vi "main elapsed time.vi"() -> ()   [LabVIEW 2019]
uses:
  Controls/Estats.ctl
panel:
  out "Numeric":i32
  in  "stop":bool
  out "Boolean":bool
  # "fixar-se en la velocitat d'execució ara"
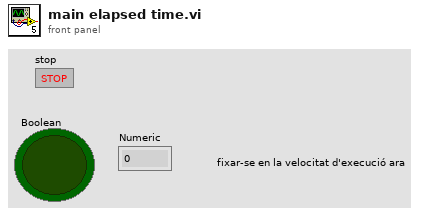
[diagram p1: front panel]
types:
  T1 = typedef "Estats.ctl" = enum16{"inicialitza", "Estat1", "Estat2"}
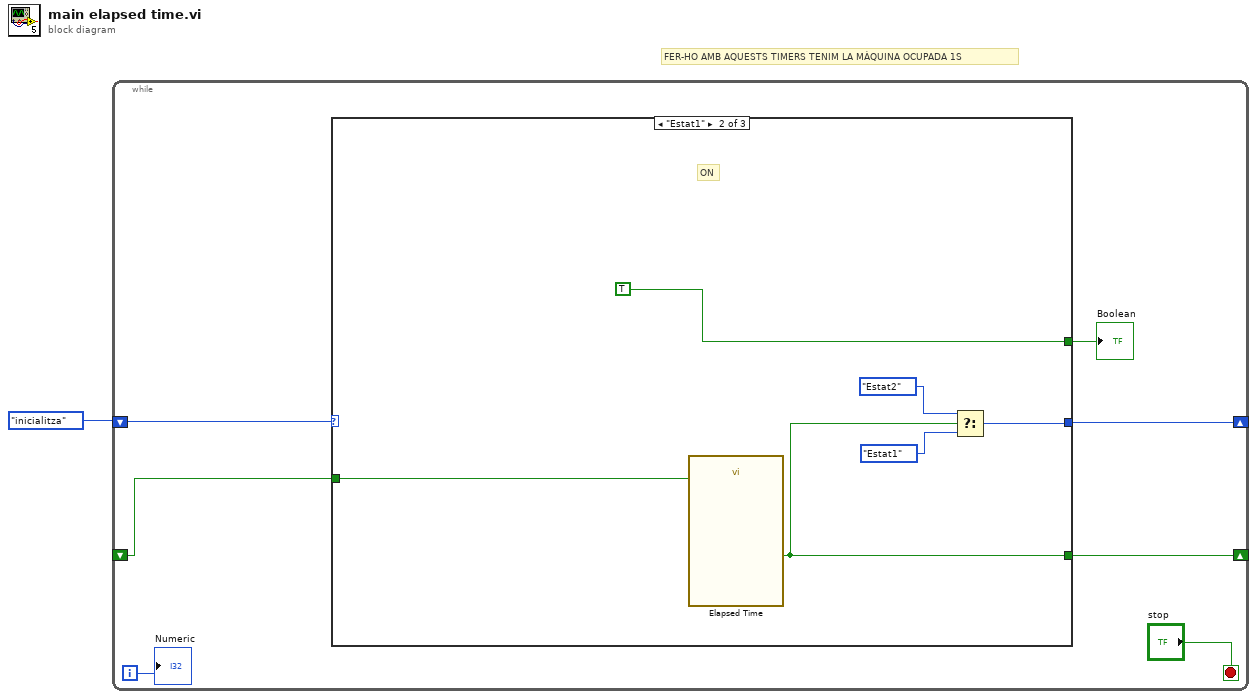
[diagram p0: block diagram]
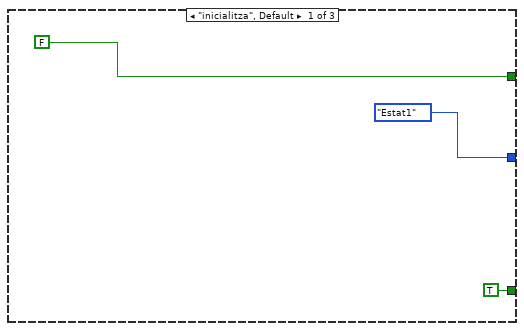
[diagram p2: hidden frame]
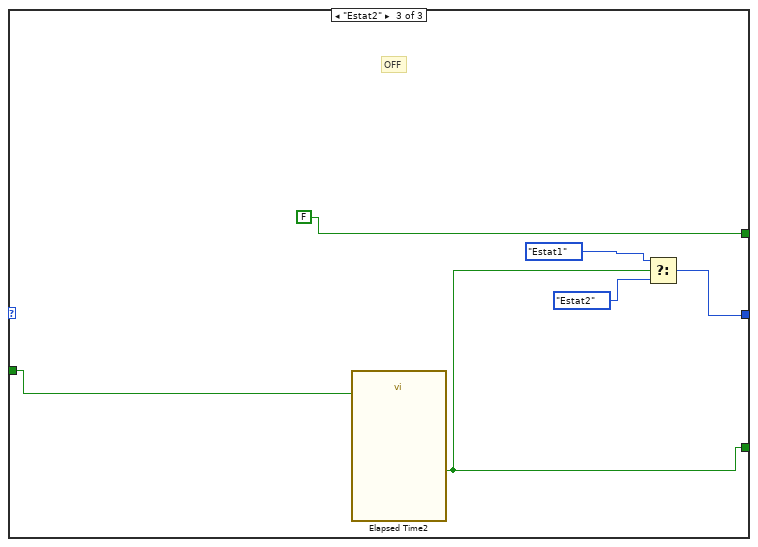
[diagram p3: hidden frame]
diagram:
  # "FER-HO AMB AQUESTS TIMERS TENIM LA MÀQUINA OCUPADA 1S"
  n1 = while {
    shift-right: [w7] -> _
    shift-left: Estats."inicialitza" ("Enum") -> [w8]
    shift-right: [w4] -> _
    shift-left: _ -> [w3]
    i -> [w2]
    stop <- "stop" stop-if-true
    n2 = case shown="\"Estat1\"" w8 {
      tunnel: [Estats."Estat1" ("Enum") w14 w22] -> w7
      tunnel: [FALSE ("Boolean") TRUE ("Boolean") FALSE ("Boolean")] -> w5
      tunnel: [TRUE ("Time has Elapsed") w13 w20] -> w4
      tunnel: w3 -> [_ w12 w19]
      frame "inicialitza", Default {
      }
      frame "Estat1" {
        # "ON"
        n3 = call "Elapsed Time"("Reset"=w12) -> ("Time has Elapsed"=w13:bool)  [unwired: 11 in, 7 out]
        n4 = Select(t=Estats."Estat2" ("Enum"), s=w13, f=Estats."Estat1" ("Enum")) -> (s? t:f=w14:T1)
      }
      frame "Estat2" {
        # "OFF"
        n5 = call "Elapsed Time2"("Reset"=w19) -> ("Time has Elapsed"=w20:bool)  [unwired: 11 in, 7 out]
        n6 = Select(t=Estats."Estat1" ("Enum"), s=w20, f=Estats."Estat2" ("Enum")) -> (s? t:f=w22:T1)
      }
    }
    "Boolean" <- w5
    "Numeric" <- w2
  }
